vi "划线.vi"(10 "Cluster":T2, 11 "引用句柄输入":T1) -> (3 "引用句柄输出":T1)   [LabVIEW 2014]
uses:
  <vilib>/vision/Image Controls.llb/IMAQ Image.ctl
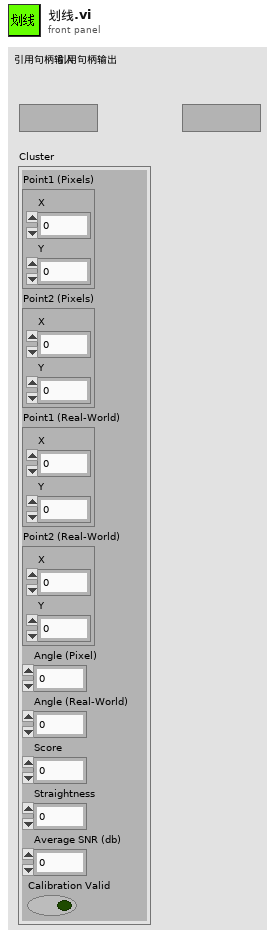
[diagram p1: front panel]
types:
  T1 = typedef "IMAQ Image.ctl" = refnum<image>
  T2 = cluster{"Point1 (Pixels)":cluster{"X":sgl, "Y":sgl}, "Point2 (Pixels)":cluster{"X":sgl, "Y":sgl}, "Point1 (Real-World)":cluster{"X":sgl, "Y":sgl}, "Point2 (Real-World)":cluster{"X":sgl, "Y":sgl}, "Angle (Pixel)":dbl, "Angle (Real-World)":dbl, "Score":dbl, "Straightness":dbl, "Average SNR (db)":dbl, "Calibration Valid":bool}
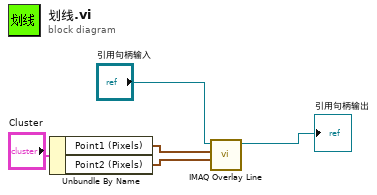
[diagram p0: block diagram]
diagram:
  n1 = Unbundle By Name("Cluster") -> ("Point1 (Pixels)"=w1:cluster{"X":sgl, "Y":sgl}, "Point2 (Pixels)"=w2:cluster{"X":sgl, "Y":sgl})
  n2 = call "IMAQ Overlay Line"("End Point"=w2, "Start Point"=w1, "Image"="引用句柄输入") -> ("Image Out"=→"引用句柄输出":T1)  [unwired: 7 in, 1 out]
